vi "Joystick to RC Override.vi"(8 "Error In":errorcluster, 11 "Aircraft ID":u8) -> (0 "Error Out":errorcluster, 3 "output cluster":T1)   [LabVIEW 2014]
uses:
  Aircraft Information/Sub VI/Get Aircraft RC.vi
  Joystick/FGVs/Joystick Input/Method VIs/Get Joystick Input.vi
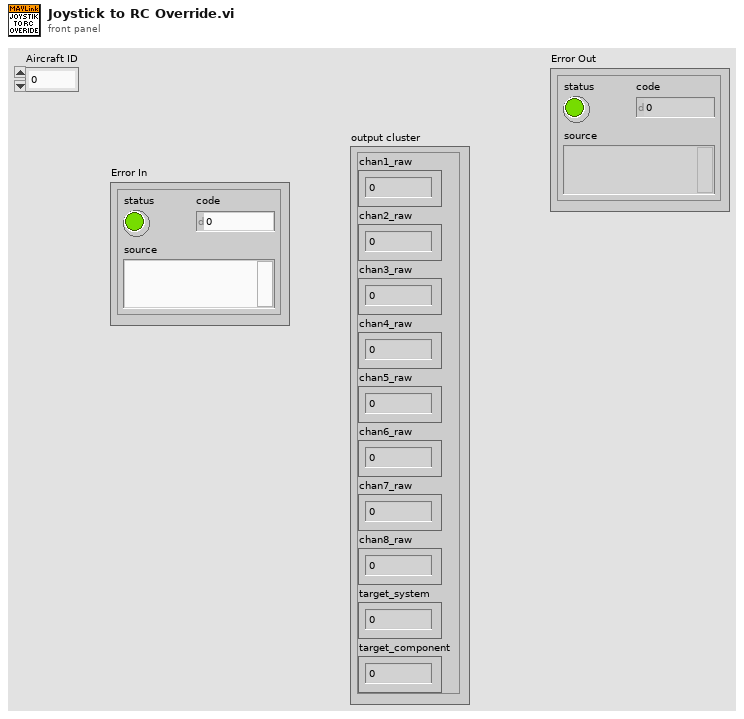
[diagram p1: front panel]
types:
  T1 = cluster{"chan1_raw":u16, "chan2_raw":u16, "chan3_raw":u16, "chan4_raw":u16, "chan5_raw":u16, "chan6_raw":u16, "chan7_raw":u16, "chan8_raw":u16, "target_system":u8, "target_component":u8}
  T2 = typedef "Joystick Input.ctl" = cluster{"Roll (%)":dbl, "Pitch (%)":dbl, "Yaw (%)":dbl, "Throttle (%)":dbl, "Brake":bool, "Emergency Stop":bool, "Arm":bool, "Disarm":bool}
  T3 = typedef "Aircraft RC Data.ctl" = cluster{"Channel 1 Min":i16, "Channel 1 Max":i16, "Channel 2 Min":i16, "Channel 2 Max":i16, "Channel 3 Min":i16, "Channel 3 Max":i16, "Channel 4 Min":i16, "Channel 4 Max":i16}
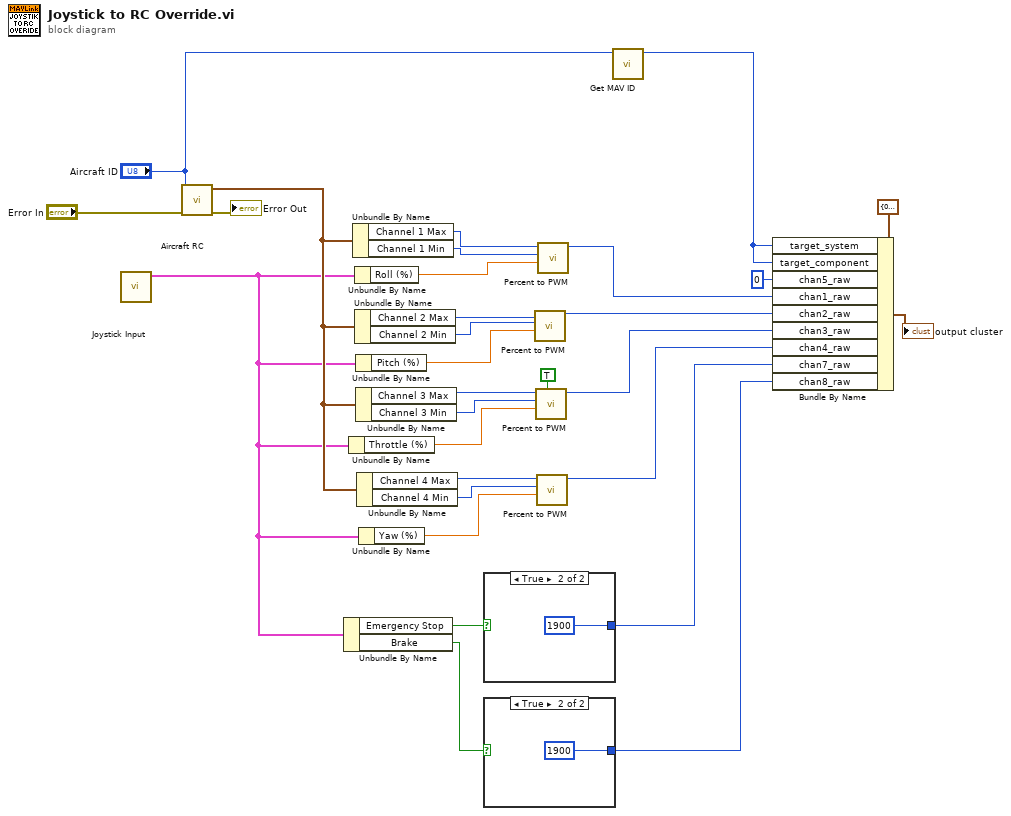
[diagram p0: block diagram]
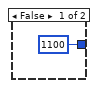
[diagram p2: hidden frame]
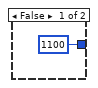
[diagram p3: hidden frame]
diagram:
  n1 = call-poly "Joystick Input.vi"() -> ("Joystick Input Out"=w4:T2)  [unwired: 11 in]
  n2 = call-poly "Aircraft RC.vi"("Error In"="Error In", "Aircraft ID"="Aircraft ID") -> ("Error Out"=→"Error Out":errorcluster, "Aircraft RC Data"=w5:T3)  [unwired: 8 in]
  n3 = Unbundle By Name(w4) -> ("Emergency Stop"=w16:bool, "Brake"=w8:bool)
  n4 = Unbundle By Name(w4) -> ("Throttle (%)"=w20:dbl)
  n5 = Unbundle By Name(w5) -> ("Channel 1 Max"=w29:i16, "Channel 1 Min"=w28:i16)
  n6 = Unbundle By Name(w4) -> ("Roll (%)"=w27:dbl)
  n7 = Unbundle By Name(w5) -> ("Channel 2 Max"=w26:i16, "Channel 2 Min"=w25:i16)
  n8 = Unbundle By Name(w4) -> ("Pitch (%)"=w24:dbl)
  n9 = Unbundle By Name(w5) -> ("Channel 3 Max"=w22:i16, "Channel 3 Min"=w21:i16)
  n10 = Unbundle By Name(w5) -> ("Channel 4 Max"=w19:i16, "Channel 4 Min"=w18:i16)
  n11 = Unbundle By Name(w4) -> ("Yaw (%)"=w17:dbl)
  n12 = case shown="True" w16 {
    tunnel: [u16 1100 u16 1900] -> w9
    frame False {
    }
    frame True {
    }
  }
  n13 = case shown="True" w8 {
    tunnel: [u16 1100 u16 1900] -> w7
    frame False {
    }
    frame True {
    }
  }
  n14 = call "Percent to PWM.vi"("Percent In"=w24, "Channel Min"=w25, "Channel Max"=w26) -> ("PWM"=w12:u16)  [unwired: 8 in]
  n15 = call "Percent to PWM.vi"("Throttle (T)/ RPY (F)"=TRUE, "Percent In"=w20, "Channel Min"=w21, "Channel Max"=w22) -> ("PWM"=w11:u16)  [unwired: 7 in]
  n16 = call "Percent to PWM.vi"("Percent In"=w17, "Channel Min"=w18, "Channel Max"=w19) -> ("PWM"=w10:u16)  [unwired: 8 in]
  n17 = call "Percent to PWM.vi"("Percent In"=w27, "Channel Min"=w28, "Channel Max"=w29) -> ("PWM"=w13:u16)  [unwired: 8 in]
  n18 = call "Get MAV ID.vi"("Aircraft Index"="Aircraft ID") -> ("Aircraft ID"=w2:u8)  [unwired: 9 in, 1 out]
  n19 = Bundle By Name(cluster=T1 {"chan1_raw"=0, "chan2_raw"=0, "chan3_raw"=0, "chan4_raw"=0, "chan5_raw"=0, "chan6_raw"=0, "chan7_raw"=0, "chan8_raw"=0, "target_system"=0, "target_component"=0} ("Payload"), "target_system"=w2, "target_component"=w2, "chan5_raw"=u16 0, "chan1_raw"=w13, "chan2_raw"=w12, "chan3_raw"=w11, "chan4_raw"=w10, "chan7_raw"=w9, "chan8_raw"=w7) -> (→"output cluster":T1)
